vi "Green Rectsv1.vi"(0 "Rectangle":T1, 1 "Margin":i32=1) -> (2 "Test Upper":i32[](array[numeric]), 3 "Test Lower":i32[](array[numeric]), 4 "Orig Upper":i32[](array[numeric]), 5 "Orig Lower":i32[](array[numeric]))   [LabVIEW 2013]
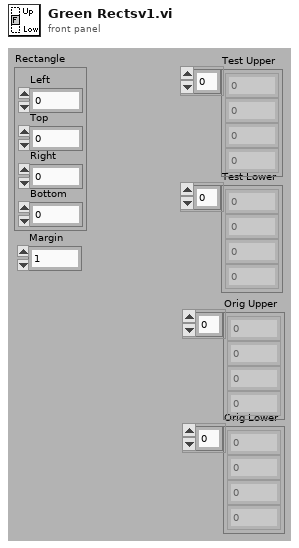
[diagram p1: front panel]
types:
  T1 = cluster{"Left":i32, "Top":i32, "Right":i32, "Bottom":i32}
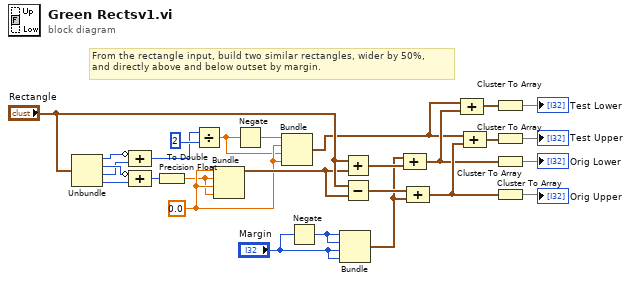
[diagram p0: block diagram]
diagram:
  w12 = 0.0
  # "From the rectangle input, build two similar rectangles, wider by 50%,\nand directly above and below outset by margin."
  n1 = Unbundle("Rectangle") -> ("Left"=w18:i32, "Top"=w26:i32, "Right"=w17:i32, "Bottom"=w27:i32)
  n2 = Compound Arithmetic op=ADD(invert w18, w17) -> (w15:i32)
  n3 = Compound Arithmetic op=ADD(invert w26, w27) -> (w14:i32)
  n4 = To Double Precision Float(number=w14) -> (double precision float=w8:dbl)
  n5 = Divide(x=w15, y=2) -> (x/y=w11:dbl)
  n6 = Bundle(w12, w8, w12, w8) -> (w23:cluster{dbl, dbl, dbl, dbl})  [unwired: 1 out]
  n7 = Negate(x=w11) -> (-x=w13:dbl)
  n8 = Bundle(w13, w12, w11, w12) -> (w5:cluster{dbl, dbl, dbl, dbl})  [unwired: 1 out]
  n9 = Negate(x="Margin") -> (-x=w10:i32)
  n10 = Bundle(w10, w10, "Margin"="Margin", "Margin"="Margin") -> (w19:cluster{i32, i32, "Margin":i32, "Margin":i32})  [unwired: 1 out]
  n11 = Add(x="Rectangle", y=w23) -> (x+y=w21:cluster{dbl, dbl, dbl, dbl})
  n12 = Subtract(x="Rectangle", y=w23) -> (x-y=w20:cluster{dbl, dbl, dbl, dbl})
  n13 = Compound Arithmetic op=ADD(w19, w21) -> (w6:cluster{dbl, dbl, dbl, dbl})
  n14 = Compound Arithmetic op=ADD(w20, w19) -> (w7:cluster{dbl, dbl, dbl, dbl})
  n15 = Compound Arithmetic op=ADD(w5, w6) -> (w4:cluster{dbl, dbl, dbl, dbl})
  n16 = Compound Arithmetic op=ADD(w5, w7) -> (w3:cluster{dbl, dbl, dbl, dbl})
  n17 = Cluster To Array(cluster=w4) -> (array=→"Test Lower":dbl[])
  n18 = Cluster To Array(cluster=w3) -> (array=→"Test Upper":dbl[])
  n19 = Cluster To Array(cluster=w6) -> (array=→"Orig Lower":dbl[])
  n20 = Cluster To Array(cluster=w7) -> (array=→"Orig Upper":dbl[])
